vi "CT_PSChargeControl.vi"(0 "Array of Power Supply Clusters":T1[](array[typedef]) caption="Power Supplies" {"Charge Voltage (kV)" format="%#_2f"; "Charge Current (A)" format="%#.2e"; "Capacitance per load" format="%#.2e"}) -> (1 "Array of Power Supply Delay and Enable":cluster{"PS Delay":dbl, "PS Enable":bool}[](array[cluster]), 2 "Longest Charge Time":dbl)   [LabVIEW 2016]
uses:
  PScluster.ctl
panel:
  out "Expected Charge Time":dbl[](array[numeric])
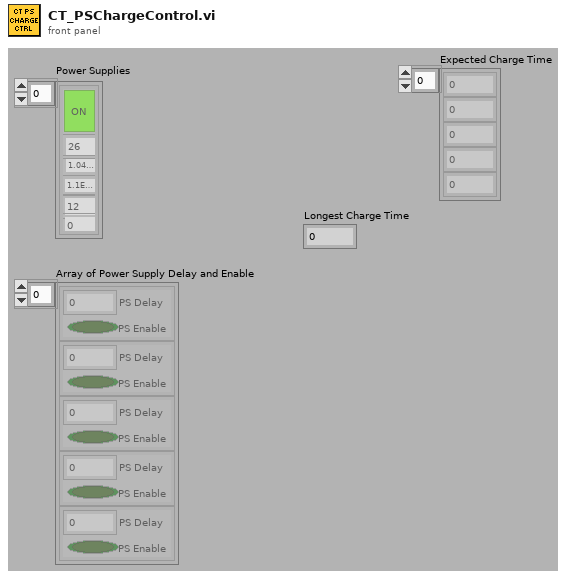
[diagram p1: front panel]
types:
  T1 = typedef "PScluster.ctl" = cluster{"On/Off Selector":bool, "Number of Loads":u32, "Capacitance per load":dbl, "Charge Current (A)":dbl, "Charge Voltage (kV)":dbl, "PWM calib":dbl}
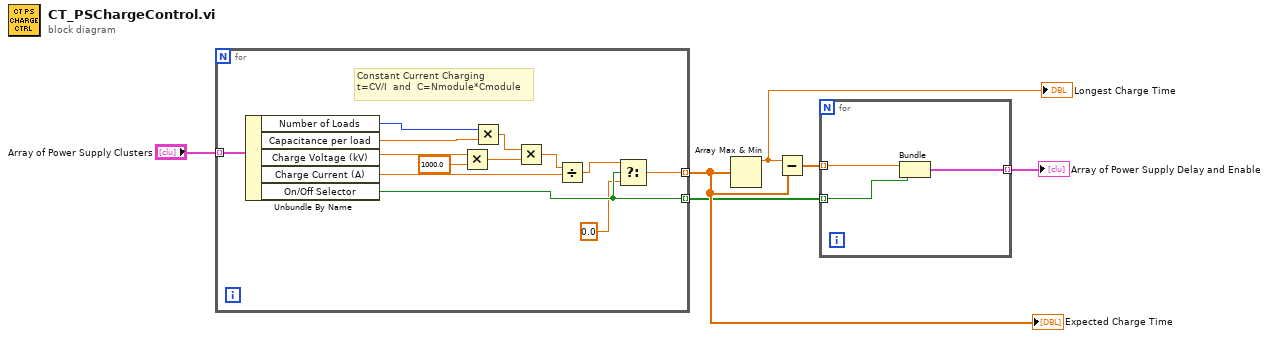
[diagram p0: block diagram]
diagram:
  n1 = for {
    tunnel: "Array of Power Supply Clusters" -> [w19] mode=indexing
    tunnel: [w9] -> w4 mode=indexing
    tunnel: [w8] -> w2 mode=indexing
    # "Constant Current Charging\nt=CV/I  and  C=Nmodule*Cmodule"
    n2 = Unbundle By Name(w19) -> ("Number of Loads"=w18:u32, "Capacitance per load"=w17:dbl, "Charge Voltage (kV)"=w13:dbl, "Charge Current (A)"=w14:dbl, "On/Off Selector"=w8:bool)
    n3 = Multiply(x=w13, y=1000.0) -> (x*y=w12:dbl)
    n4 = Multiply(x=w18, y=w17) -> (x*y=w16:dbl)
    n5 = Multiply(x=w16, y=w12) -> (x*y=w15:dbl)
    n6 = Divide(x=w15, y=w14) -> (x/y=w10:dbl)
    n7 = Select(t=w10, s=w8, f=0.0) -> (s? t:f=w9:dbl)
  }
  "Expected Charge Time" <- w4
  n8 = Array Max & Min(array=w4) -> (max value=w5:dbl)  [unwired: 3 out]
  "Longest Charge Time" <- w5
  n9 = Subtract(x=w5, y=w4) -> (x-y=w3:dbl[])
  n10 = for {
    tunnel: w3 -> [w22] mode=indexing
    tunnel: w2 -> [w21] mode=indexing
    tunnel: [w20] -> w1 mode=indexing
    n11 = Bundle(w22, "On/Off Selector"=w21) -> (w20:cluster{dbl, "On/Off Selector":bool})  [unwired: 1 in]
  }
  "Array of Power Supply Delay and Enable" <- w1
